vi "Assemble WRITE PDU (u16).vi"(1 "u16 value":u16=1 format="%04x", 2 "Register":T1 items=["Control"=0, "RPM set-point"=4, "Drive status"=5, "Output RPM"=6, "Motor current"=7, "Motor torque"=8, "Motor power"=9, "DC bus voltage"=22, "Drive power stage temperature"=23, "kWh meter"=31, "MWh meter"=32, "Running time - hours"=33, "Running time - seconds"=34, "Drive internal temperature"=38, "Motor RMS voltage"=42, "Extended drive status"=2000], 3 "Drive address":T2=1 items=["0", "1", "2", "3", "4", "5", "6", "7", "8", "9", "10", "11", "12", "13", "14", "15", "16", "17", "18", "19", "20", "21", "22", "23", "24", "25", "26", "27", "28", "29", "30", "31", "32", "33", "34", "35", "36", "37", "38", "39", "40", "41", "42", "43", "44", "45", "46", "47", "48", "49", "50", "51", "52", "53", "54", "55", "56", "57", "58", "59", "60", "61", "62", "63"]) -> (0 "Ser out string":string)   [LabVIEW 2020]
doc: "Modbus RTU for Invertek drives. Paul Nathan 19-JUN-2022."
uses:
  ctls/Drive address.ctl
  ctls/Register.ctl
  ctls/Write PDU (u16).ctl
  ctls/Function.ctl
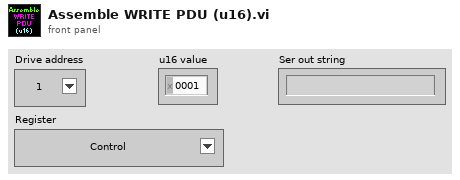
[diagram p1: front panel]
types:
  T1 = typedef "Register.ctl" = u16
  T2 = typedef "Drive address.ctl" = u8
  T3 = typedef "Function.ctl" = u8
  T4 = typedef "Write PDU (u16).ctl" = cluster{"Drive address":T2, "Function":T3, "Register":T1, "u16 value":u16}
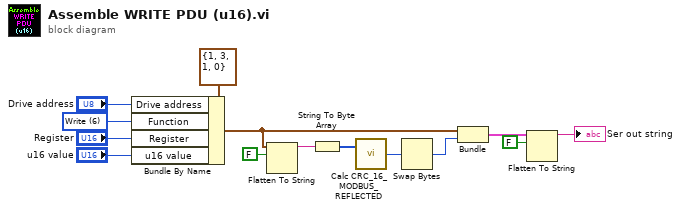
[diagram p0: block diagram]
diagram:
  w1 = T3 6 items=["Read"=3, "Write"=6] ("Function")
  n1 = Bundle By Name(cluster=T4 {"Drive address"=1, "Function"=3, "Register"=1, "u16 value"=0} ("Read PDU"), "Drive address"="Drive address", "Function"=w1, "Register"="Register", "u16 value"="u16 value") -> (w8:T4)
  n2 = Flatten To String(anything=w8, prepend array or string size? (T)=FALSE) -> (data string=w10:string)  [unwired: 2 in, 2 out]
  n3 = String To Byte Array(string=w10) -> (unsigned byte array=w9:u8[])
  n4 = call "Calc CRC_16_MODBUS_REFLECTED.vi"("Data bytes"=w9) -> ("CRC_16-MODBUS"=w7:u16)  [unwired: 1 in]
  n5 = Swap Bytes(anything=w7) -> (byte swapped=w5:u16)
  n6 = Bundle("Read PDU"=w8, w5) -> (w4:cluster{"Read PDU":T4, u16})  [unwired: 1 in]
  n7 = Flatten To String(anything=w4, prepend array or string size? (T)=FALSE) -> (data string=→"Ser out string":string)  [unwired: 2 in, 2 out]
